vi "Remove Song From Queue by Index.vi"(8 "error in (no error)":errorcluster, 10 "Index":u32, 11 "SongQueueActor In":refnum<class "SongQueueActor.lvclass">) -> (0 "error out":errorcluster, 3 "SongQueueActor Out":refnum<class "SongQueueActor.lvclass">)   [LabVIEW 2015, in "SongQueueActor.lvlib" / "SongQueueActor.lvclass"]
uses:
  SongQueueActor.lvclass
  SongQueueActor.lvclass/SongQueueActor.ctl
  builds/xctls/Song Queue/Song Queue.lvlibp/app/controls/Queue Song Display.ctl
  builds/xctls/Song Queue/Song Queue.lvlibp/file/MusicElement/Song/Song Duration.ctl
  builds/xctls/Song Queue/Song Queue.lvlibp/app/controls/Dequeue Control.ctl
  builds/xctls/Song Queue/Song Queue.lvlibp/app/xctls/SongQueue/Song Queue.xctl
  file/MusicElement/MusicElementLibrary/MusicElementLibrary.lvclass
  builds/xctls/Song Queue/Song Queue.lvlibp
  builds/xctls/Song Queue/Song Queue.lvlibp/file/MusicElement/Song/Song.lvclass
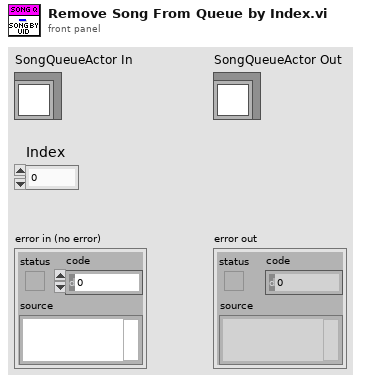
[diagram p1: front panel]
types:
  T1 = typedef "Song Queue.lvlibp/Queue Song Display.ctl" = cluster{"Song Name":string, "Artist":string, "Album":string, "Duration (s)":T2, "UID":string, "Dequeue":T3}
  T2 = typedef "Song Queue.lvlibp/Song.lvclass/Song Duration.ctl" = timestamp
  T3 = typedef "Song Queue.lvlibp/Dequeue Control.ctl" = bool
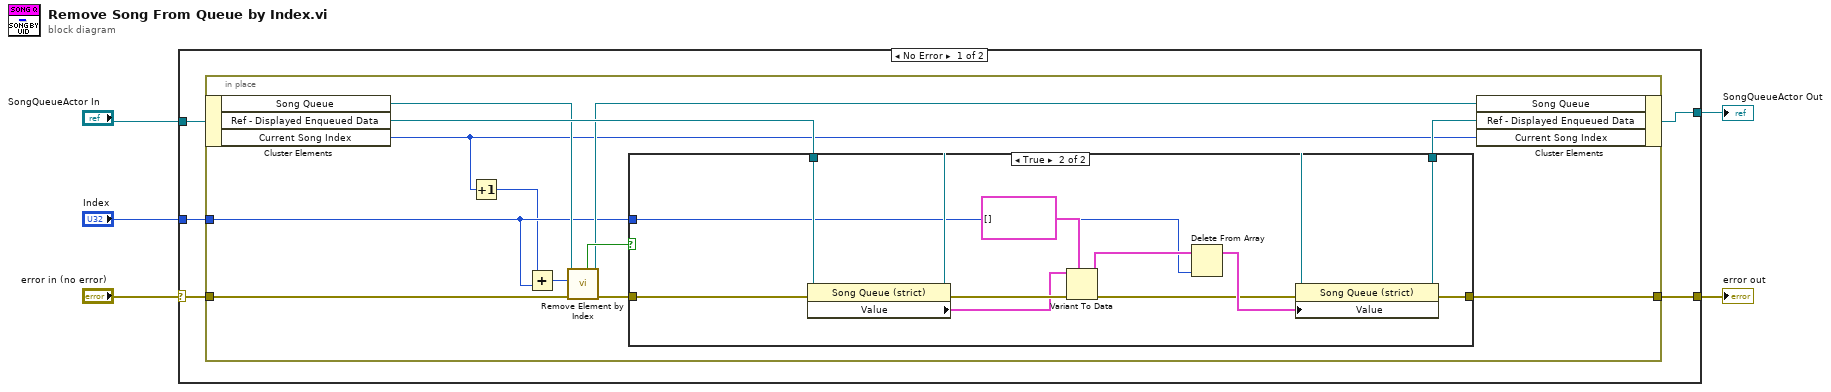
[diagram p0: block diagram]
diagram:
  n1 = case shown="No Error" "error in (no error)" {
    selector: "error in (no error)" -> [w9 w38]
    tunnel: [w7 w38] -> w4
    tunnel: [w8 w37] -> w3
    tunnel: "SongQueueActor In" -> [w10 w37]
    tunnel: "Index" -> [w6 _]
    frame No Error {
      n2 = in-place {
        in-place-border: w9 -> [w18]
        in-place-border: [w21] -> w7
        in-place-border: w6 -> [w12]
        n3 = in-place-cluster #1(w10) -> ("Song Queue"=w14:refnum<class "SongLibrary.lvclass">, "Ref - Displayed Enqueued Data"=w22:refnum<vi>, "Current Song Index"=w13:i32)
        n4 = Increment(x=w13) -> (x+1=w11:i32)
        n5 = Add(x=w11, y=w12) -> (x+y=w16:u32)
        n6 = call "Remove Element by Index.vi"("error in (no error)"=w18, "Index"=w16, "MusicElementLibrary"=w14) -> ("error out"=w19:errorcluster, "MusicElementLibrary"=w15:refnum<class "SongLibrary.lvclass">, "Removed?"=w17:bool)  [unwired: 6 in]
        n7 = case shown="True" w17 {
          tunnel: w22 -> [w24 w36]
          tunnel: [w23 w31] -> w21
          tunnel: [w24 w30] -> w20
          tunnel: w19 -> [w23 w26]
          tunnel: w12 -> [_ w25]
          frame False {
          }
          frame True {
            n8 = property class="Song Queue (strict)"(reference=w36, error in=w26) -> (reference out=w34:refnum<vi>, error out=w35:errorcluster, "Value"=w27:T1[])
            n9 = Variant To Data(error in=w35, type=T1[] [] ("Song Queue"), Variant=w27) -> (data=w33:T1[], error out=w29:errorcluster)
            n10 = Delete From Array(array=w33, index=w25) -> (array with subset deleted=w32:T1[])  [unwired: 1 in, 1 out]
            n11 = property class="Song Queue (strict)"(reference=w34, error in=w29, "Value"=w32) -> (reference out=w30:refnum<vi>, error out=w31:errorcluster)
          }
        }
        n12 = in-place-cluster #1("Song Queue"=w15, "Ref - Displayed Enqueued Data"=w20, "Current Song Index"=w13) -> (w8:refnum<class "SongQueueActor.lvclass">)
      }
    }
    frame Error {
    }
  }
  "error out" <- w4
  "SongQueueActor Out" <- w3
